vi "SRV_0xdddd String to Sensor View Indicator Name.vi"(7 "dddd":string, 11 "error in (no error)":errorcluster) -> (8 "Sensor View Indicator Names":T1, 15 "error out":errorcluster)   [LabVIEW 2014]
uses:
  SRV_Sensors Names.ctl
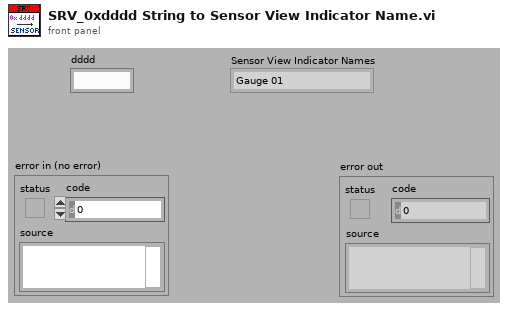
[diagram p1: front panel]
types:
  T1 = typedef "SRV_Sensors Names.ctl" = enum16{"Gauge 01", "Gauge 02", "Gauge 03", "Gauge 04", "Meter 01", "Meter 02", "Meter 03", "Meter 04", "Numeric 01", "Numeric 02", "Numeric 03", "Numeric 04", "Numeric 05", "Numeric 06", "Numeric 07", "Numeric 08", "Boolean 01", "Boolean 02", "Boolean 03", "Boolean 04", "Boolean 05", "Boolean 06", "Boolean 07", "Boolean 08", "Boolean 09", "Boolean 10", "Boolean 11", "Boolean 12", "Boolean 13", "Boolean 14", "Boolean 15", "Boolean 16", "Boolean 17", "Boolean 18", "Boolean 19", "Boolean 20", "Boolean 21", "Boolean 22", "Boolean 23", "Boolean 24", "Boolean 25", "Boolean 26", "Boolean 27", "Boolean 28", "Boolean 29", "Boolean 30", "Boolean 31", "Boolean 32"}
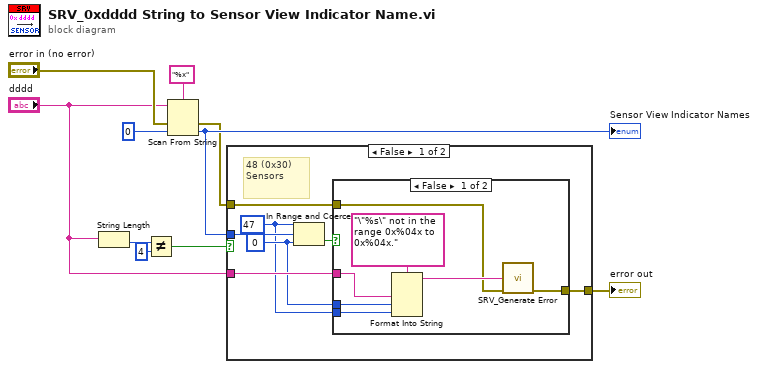
[diagram p0: block diagram]
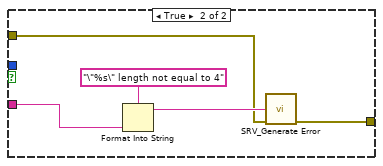
[diagram p3: hidden frame]
diagram:
  n1 = String Length(string="dddd") -> (length=w8:i32)
  n2 = Not Equal?(x=w8, y=4) -> (x != y?=w5:bool)
  n3 = Scan From String(format string="%x", input string="dddd", error in="error in (no error)", default 1=u16 0) -> (error out=w1:errorcluster, output 1=w2:u16)  [unwired: 1 in, 2 out]
  "Sensor View Indicator Names" <- w2
  n4 = case shown="False" w5 {
    tunnel: [w15 w30] -> w6
    tunnel: "dddd" -> [w13 w28]
    tunnel: w2 -> [w17 _]
    tunnel: w1 -> [w16 w26]
    frame False {
      w11 = u16 47 ("upper limit")
      w12 = u16 0 ("lower limit")
      # "48 (0x30) Sensors"
      n5 = In Range and Coerce(upper limit=w11, x=w17, lower limit=w12) -> (In Range?=w14:bool)  [unwired: 1 out]
      n6 = case shown="False" w14 {
        tunnel: w16 -> [w20 w25]
        tunnel: [w24 w25] -> w15
        tunnel: w13 -> [w23 _]
        tunnel: w12 -> [w19 _]
        tunnel: w11 -> [w18 _]
        frame False {
          n7 = Format Into String(format string="\"%s\" not in the range 0x%04x to 0x%04x.", w23, w19, w18) -> (resulting string=w22:string)  [unwired: 2 in, 1 out]
          n8 = call "SRV_Generate Error.vi"("Message"=w22, "error in (no error)"=w20) -> ("error out"=w24:errorcluster)  [unwired: 13 in]
        }
        frame True {
        }
      }
    }
    frame True {
      n9 = Format Into String(format string="\"%s\" length not equal to 4", w28) -> (resulting string=w27:string)  [unwired: 2 in, 1 out]
      n10 = call "SRV_Generate Error.vi"("Message"=w27, "error in (no error)"=w26) -> ("error out"=w30:errorcluster)  [unwired: 13 in]
    }
  }
  "error out" <- w6
